vi "Periodic Tasks.vi"   [LabVIEW 2019]
doc: "This VI runs in parallel to other tasks. It can contain as many user-defined periodic loops as you need. These can carry out PID or other sorts of timed response."
uses:
  <vilib>/Rock Robotics/WPI/Utilities/WPI_GetSetVariantRefNum.vi
  <vilib>/Utility/config.llb/Write Key (Double).vi
  <vilib>/Utility/config.llb/NI_LVConfig.lvlib
types:
  T1 = typedef "WPI_JoystickDevRef.ctl" = cluster{"Device":T2}
  T2 = typedef "WPI_JoystickDeviceEnum.ctl" = enum16{"USB 0", "USB 1", "USB 2", "USB 3", "USB 4", "USB 5"}
  T3 = typedef "Color Sensor V3 DevRef.ctl" = cluster{"I2CDevRef":T4}
  T4 = typedef "WPI_I2CDevRef.ctl" = cluster{"DevStatus":errorcluster, "Device Address":u8, "Handle":i32, "I2C Bus":T5}
  T5 = typedef "i2c_bus.ctl" = enum16{"I2C On-Board", "I2C MXP", "Invalid"}
  T6 = typedef "NI_LVConfig.lvlib/Config Data RefNum.ctl" = refnum<k1>
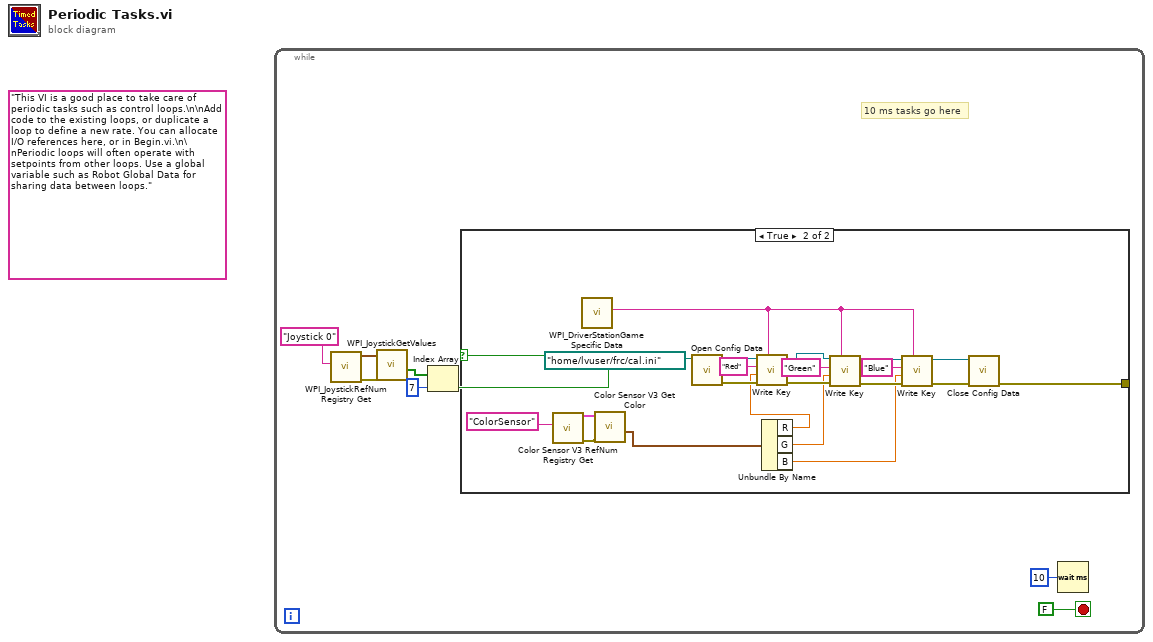
[diagram p0: block diagram]
diagram:
  (unwired) "This VI is a good place to take care of periodic tasks such as control loops.\n\nAdd code to the existing loops, or duplicate a loop to define a new rate. You can allocate I/O references here, or in Begin.vi.\n\nPeriodic loops will often operate with setpoints from other loops. Use a global variable such as Robot Global Data for sharing data between loops."
  n1 = while {
    stop <- FALSE stop-if-true
    # "10 ms tasks go here"
    n2 = call <vilib>:"WPI_JoystickRefNum Registry Get.vi"("refnum name"="Joystick 0") -> ("error out"=w4:errorcluster, "JoystickDevRef"=w5:T1)  [unwired: 9 in]
    n3 = call <vilib>:"WPI_JoystickGetValues.vi"("error in (no error)"=w4, "JoystickDevRef"=w5) -> ("Buttons"=w3:bool[])  [unwired: 5 in, 4 out]
    n4 = Index Array(array=w3, index=7) -> (element=w1:bool)
    n5 = case shown="True" w1 {
      tunnel: [_ w16] -> _
      frame False {
      }
      frame True {
        n6 = call <vilib>:"Color Sensor V3 RefNum Registry Get.vi"("refnum name"="ColorSensor") -> ("error out"=w13:errorcluster, "ColorSensorDevRef"=w14:T3)  [unwired: 9 in]
        n7 = call <vilib>:"WPI_DriverStationGame Specific Data.vi"() -> ("Game Specific Data"=w19:string)  [unwired: 11 in]
        n8 = call <vilib>:"Color Sensor V3 Get Color.vi"("error in (no error)"=w13, "ColorSensorDevRef"=w14) -> ("Normalized Color"=w12:cluster{"R":dbl, "G":dbl, "B":dbl})  [unwired: 6 in, 3 out]
        n9 = call <vilib>:"Open Config Data.vi"("configuration file path"=path "/home/lvuser/frc/cal.ini") -> ("error out"=w27:errorcluster, "refnum"=w28:T6)  [unwired: 8 in, 1 out]
        n10 = Unbundle By Name(w12) -> ("R"=w11:dbl, "G"=w10:dbl, "B"=w9:dbl)
        n11 = call-poly <vilib>:"Write Key.vi"("section"=w19, "error in (no error)"=w27, "value"=w11, "key"="Red", "refnum"=w28) -> ("error out"=w23:errorcluster, "refnum out"=w24:T6)  [unwired: 4 in, 1 out]
        n12 = call-poly <vilib>:"Write Key.vi"("section"=w19, "error in (no error)"=w23, "value"=w10, "key"="Green", "refnum"=w24) -> ("error out"=w22:errorcluster, "refnum out"=w21:T6)  [unwired: 4 in, 1 out]
        n13 = call-poly <vilib>:"Write Key.vi"("section"=w19, "error in (no error)"=w22, "value"=w9, "key"="Blue", "refnum"=w21) -> ("error out"=w18:errorcluster, "refnum out"=w17:T6)  [unwired: 4 in, 1 out]
        n14 = call <vilib>:"Close Config Data.vi"("error in (no error)"=w18, "refnum"=w17) -> ("error out"=w16:errorcluster)  [unwired: 8 in, 1 out]
      }
    }
    n15 = Wait (ms)(milliseconds to wait=u32 10) -> ()  [unwired: 1 out]
  }
